vi "W9EO82,FBO8PP_2 .vi"() -> ()   [LabVIEW 2021]
panel:
  out "String":string
  in  "Slide":i32(slide) scale=0.0..2.0
  out "Eredmény":dbl
  in  "Numeric":dbl
  out "gomb":bool
  in  "kapcsoló":bool
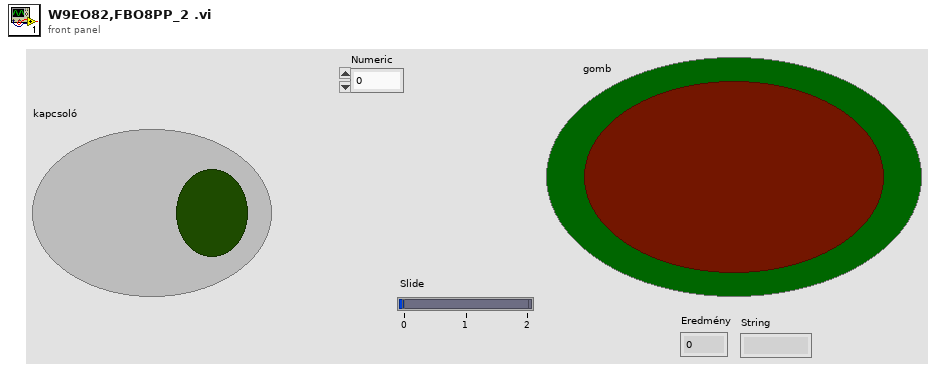
[diagram p1: front panel]
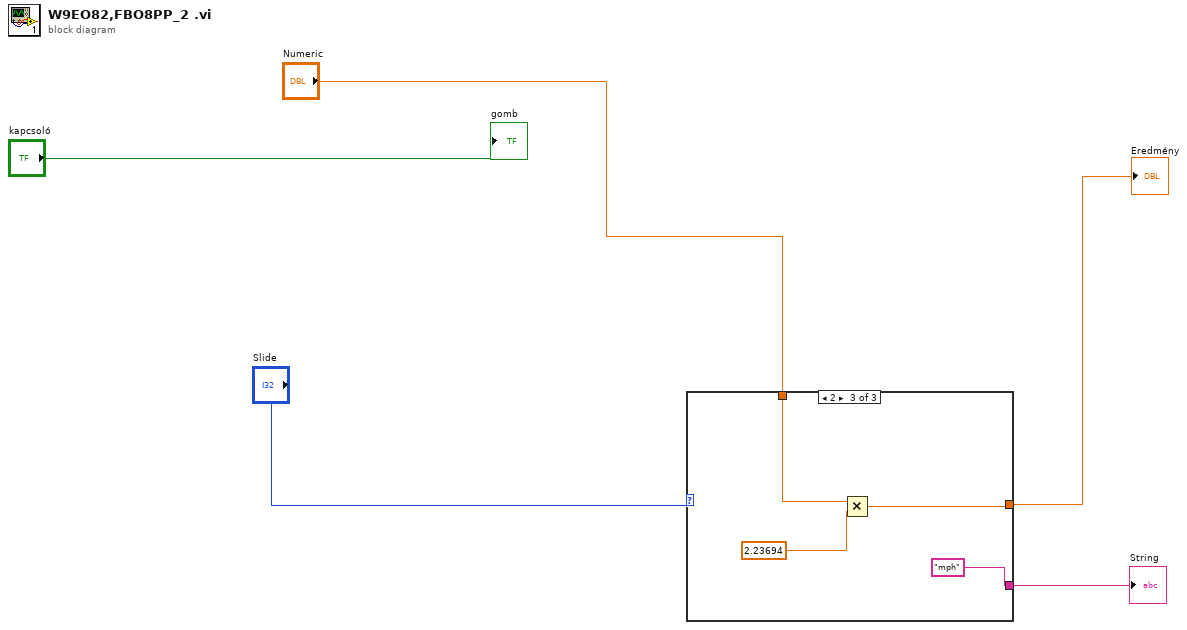
[diagram p0: block diagram]
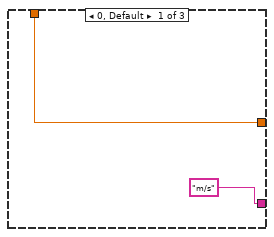
[diagram p2: hidden frame]
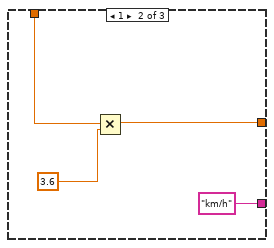
[diagram p3: hidden frame]
diagram:
  n1 = case shown="2" "Slide" {
    tunnel: "Numeric" -> [w7 w10 w14]
    tunnel: [w7 w11 w13] -> w2
    tunnel: ["m/s" "km/h" "mph"] -> w1
    frame 0, Default {
    }
    frame 1 {
      n2 = Multiply(x=w10, y=3.6) -> (x*y=w11:dbl)
    }
    frame 2 {
      n3 = Multiply(x=w14, y=2.23694) -> (x*y=w13:dbl)
    }
  }
  "Eredmény" <- w2
  "String" <- w1
  "gomb" <- "kapcsoló"
